vi "Console_CleanUp.vi"(8 "Error In":errorcluster) -> (0 "Error Out":errorcluster)   [LabVIEW 2020, in "Console.lvclass"]
uses:
  Console.lvclass
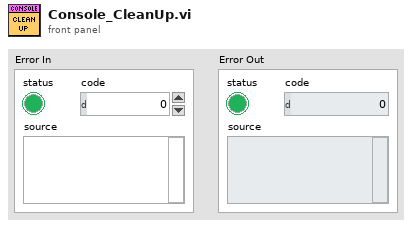
[diagram p1: front panel]
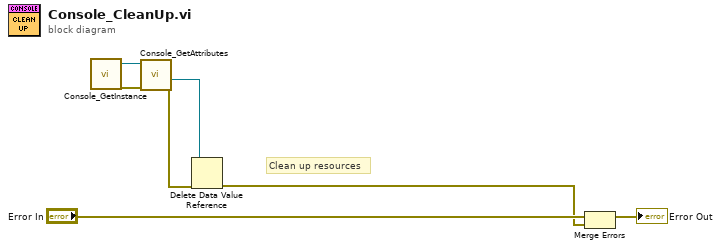
[diagram p0: block diagram]
diagram:
  # "Clean up resources"
  n1 = call "Console_GetInstance.vi"() -> ("error out"=w6:errorcluster, "reference out"=w5:refnum<class "Console.lvclass">)  [unwired: 7 in, 3 out]
  n2 = call "Console_GetAttributes.vi"("error in (no error)"=w6, "reference in"=w5) -> ("error out"=w4:errorcluster, "DataRef"=w3:refnum<data-value>)  [unwired: 6 in, 2 out]
  n3 = Delete Data Value Reference(data value reference=w3, error in=w4) -> (error out=w1:errorcluster)  [unwired: 1 out]
  n4 = Merge Errors("Error In", w1) -> (→"Error Out":errorcluster)
